vi "SIM Rosenbrock error.vi"(7 "Ros data":T1, 8 "step size":dbl, 9 "F2":dbl[](array[numeric])) -> (2 "error":dbl[](array[numeric]), 3 "F2 out":dbl[](array[numeric]))   [LabVIEW 2020]
uses:
  SIM Rosenbrock data.ctl
  SIM Factored Matrix.ctl
  SIM Ros stages.ctl
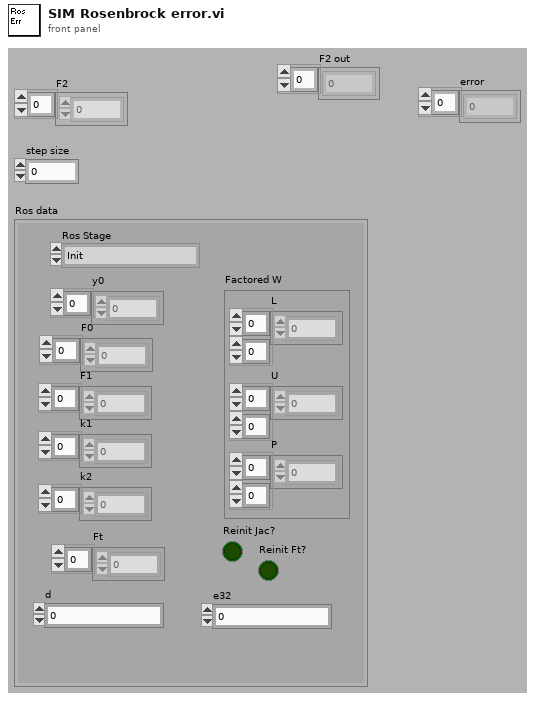
[diagram p1: front panel]
types:
  T1 = typedef "SIM Rosenbrock data.ctl" = cluster{"y0":dbl[], "F0":dbl[], "F1":dbl[], "k1":dbl[], "k2":dbl[], "Factored W":T2, "Ros Stage":T3, "Ft":dbl[], "Reinit Jac?":bool, "Reinit Ft?":bool, "d":dbl, "e32":dbl}
  T2 = typedef "SIM Factored Matrix.ctl" = cluster{"L":dbl[][], "U":dbl[][], "P":i32[][]}
  T3 = typedef "SIM Ros stages.ctl" = enum16{"Init", "Compute Jacobian", "Compute Ft", "Compute k1", "Compute k2", "Eval Error", "Choose StepSize", "Reset Integrator"}
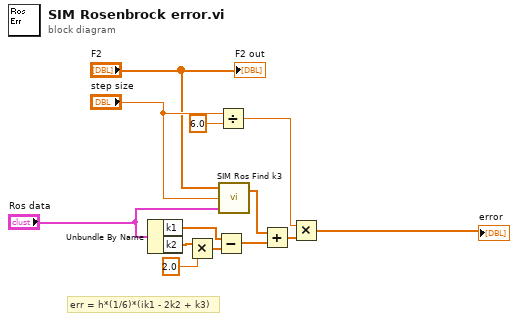
[diagram p0: block diagram]
diagram:
  # "err = h*(1/6)*(ik1 - 2k2 + k3)"
  n1 = Unbundle By Name("Ros data") -> ("k1"=w6:dbl[], "k2"=w4:dbl[])
  n2 = Multiply(x=w4, y=2.0) -> (x*y=w5:dbl[])
  n3 = Subtract(x=w6, y=w5) -> (x-y=w7:dbl[])
  n4 = Divide(x="step size", y=6.0) -> (x/y=w12:dbl)
  n5 = call "SIM Ros Find k3.vi"("Ros data"="Ros data", "step size"="step size", "F2"="F2") -> ("k"=w8:dbl[])  [unwired: 1 out]
  n6 = Add(x=w8, y=w7) -> (x+y=w11:dbl[])
  n7 = Multiply(x=w12, y=w11) -> (x*y=→"error":dbl[])
  "F2 out" <- "F2"
